vi "Set configuration chain.vi"(8 "error in (no error)":errorcluster, 9 "class names":string[](array[string]), 10 "configuration":variant[](array[variant]), 11 "Retiga in":refnum<class "Retiga.lvclass">) -> (0 "error out":errorcluster, 3 "Retiga out":refnum<class "Retiga.lvclass">)   [LabVIEW 2012, in "Retiga.lvclass"]
uses:
  Retiga.lvclass
  <vilib>/Distrio/Murmex/Murmex/Murmex.lvclass
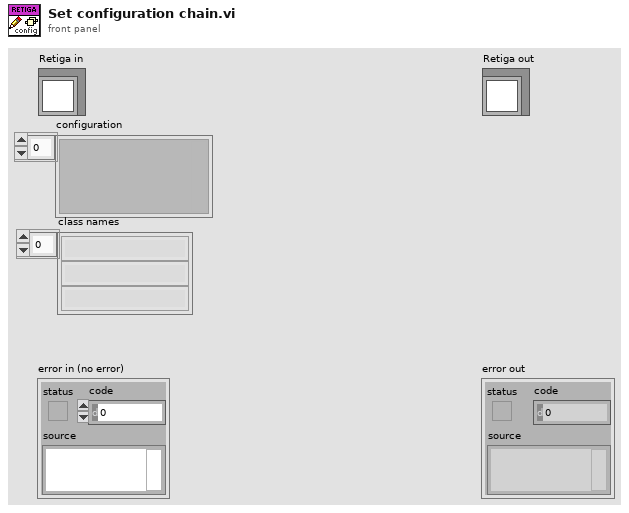
[diagram p1: front panel]
types:
  T1 = typedef "Retiga.lvclass/configuration.ctl" = cluster{"temperature":dbl, "stage component":string, "micron equivalent of pixel":dbl[unit], "max x pixel displacement":dbl, "min x pixel displacement":dbl, "max pixel discrepancy":dbl, "max y pixel displacement":dbl, "min y pixel displacement":dbl, "brightness threshold":sgl}
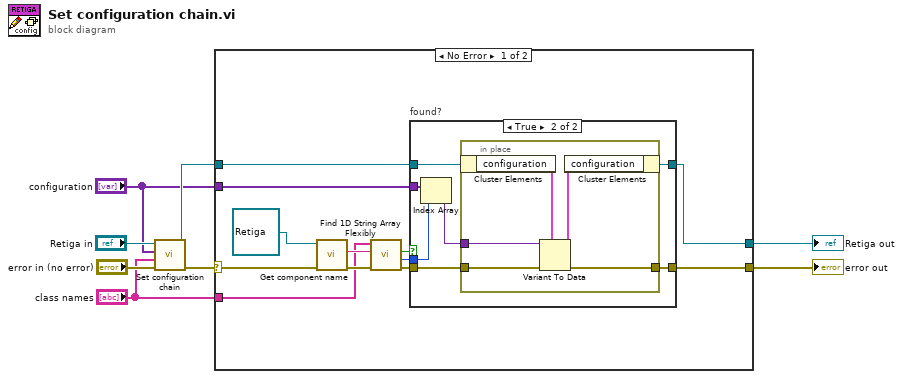
[diagram p0: block diagram]
diagram:
  n1 = call-parent "Set configuration chain.vi"("error in (no error)"="error in (no error)", "class names"="class names", "configuration"="configuration", "Murmex in"="Retiga in") -> ("error out"=w6:errorcluster, "Murmex out"=w5:refnum<class "Retiga.lvclass">)  [unwired: 6 in]
  n2 = case shown="No Error" w6 {
    selector: w6 -> [w15 w35]
    tunnel: w5 -> [w14 w36]
    tunnel: "configuration" -> [w13 _]
    tunnel: "class names" -> [w12 _]
    tunnel: [w10 w35] -> w2
    tunnel: [w9 w36] -> w1
    frame No Error {
      n3 = call <vilib>:"Get component name.vi"("error in (no error)"=w15, "Murmex in"=refnum<class "Retiga.lvclass"> refnum ("Retiga in")) -> ("error out"=w20:errorcluster, "component name"=w19:string)  [unwired: 7 in, 1 out]
      n4 = call <vilib>:"Find 1D String Array Flexibly.vi"("error in (no error)"=w20, "element"=w19, "array"=w12) -> ("error out"=w18:errorcluster, "index of element"=w16:i32, "found?"=w17:bool)  [unwired: 6 in]
      n5 = case "found?" shown="True" w17 {
        tunnel: w13 -> [_ w29]
        tunnel: w14 -> [w22 w27]
        tunnel: [w22 w26] -> w9
        tunnel: [w21 w25] -> w10
        tunnel: w18 -> [w21 w24]
        tunnel: w16 -> [_ w23]
        frame False {
        }
        frame True {
          n6 = Index Array(array=w29, index=w23) -> (element=w28:variant)
          n7 = in-place {
            in-place-border: w28 -> [w34]
            in-place-border: w24 -> [w32]
            in-place-border: [w30] -> w25
            n8 = in-place-cluster #1(w27) -> ("configuration"=w33:T1)
            n9 = Variant To Data(error in=w32, type=w33, Variant=w34) -> (data=w31:T1, error out=w30:errorcluster)
            n10 = in-place-cluster #1("configuration"=w31) -> (w26:refnum<class "Retiga.lvclass">)
          }
        }
      }
    }
    frame Error {
    }
  }
  "error out" <- w2
  "Retiga out" <- w1
